vi "ti2_setLightPath.vi"(8 "error in (no error)":errorcluster, 11 "Light Path":T1=1 items=["Eyepieces"=1, "Right"=2, "Bottom"=3, "Left"=4]) -> (0 "error out":errorcluster)   [LabVIEW 2022 SP3, in "ti2lv.lvlib"]
uses:
  ti2lv.lvlib
  ti2_lightPath.ctl
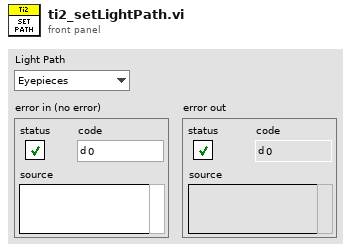
[diagram p1: front panel]
types:
  T1 = typedef "ti2lv.lvlib/ti2_lightPath.ctl" = i32
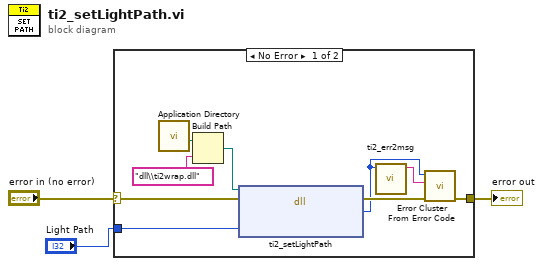
[diagram p0: block diagram]
diagram:
  n1 = case shown="No Error" "error in (no error)" {
    selector: "error in (no error)" -> [w11 w13]
    tunnel: [w12 w13] -> w3
    tunnel: "Light Path" -> [w7 _]
    frame No Error {
      n2 = call <vilib>:"Application Directory.vi"() -> ("Application Directory"=w5:path)
      n3 = Build Path(base path=w5, name or relative path="dll\\ti2wrap.dll") -> (appended path=w4:path)
      n4 = dll-call lib="?" fn="ti2_setLightPath"(path in=w4, error in=w11, "lightPath"=w7) -> (error out=w10:errorcluster, "return type"=w9:i32)  [unwired: 2 in, 1 out]
      n5 = call "ti2_err2msg.vi"("Error Code"=w9) -> ("Error Message"=w8:string)  [unwired: 10 in]
      n6 = call <vilib>:"Error Cluster From Error Code.vi"("error in (no error)"=w10, "error message (\"\")"=w8, "error code (0)"=w9) -> ("error out"=w12:errorcluster)  [unwired: 6 in]
    }
    frame Error {
    }
  }
  "error out" <- w3
